vi "Configure.vi"(8 "error in":errorcluster, 10 "ConfigRef In":T1, 11 "HH802U in":refnum<class "HH802U.lvclass">) -> (0 "error out":errorcluster, 3 "HH802U out":refnum<class "HH802U.lvclass">)   [LabVIEW 2015, in "HH802U.lvclass"]
uses:
  HH802U.lvclass
  <vilib>/Utility/config.llb/Config Data RefNum.ctl
  HH802U.lvclass/HH802U.ctl
  <vilib>/Utility/config.llb/Read Key (String).vi
  <vilib>/Utility/config.llb/Read Key (U32).vi
  <vilib>/Instr/_visa.llb/VISA Configure Serial Port (Instr).vi
  <vilib>/Utility/config.llb/NI_LVConfig.lvlib
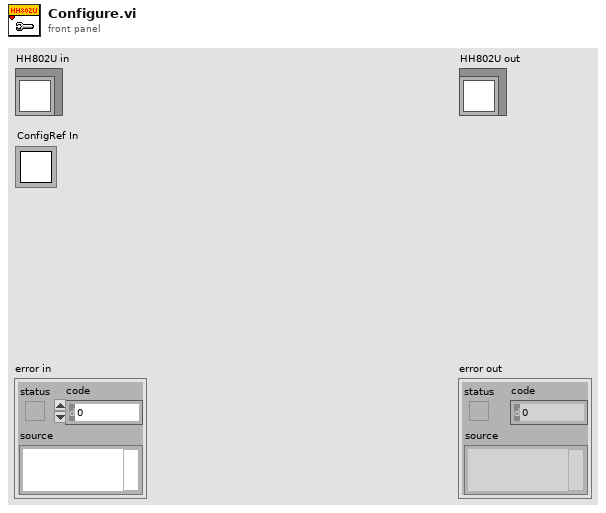
[diagram p1: front panel]
types:
  T1 = typedef "NI_LVConfig.lvlib/Config Data RefNum.ctl" = refnum<k1>
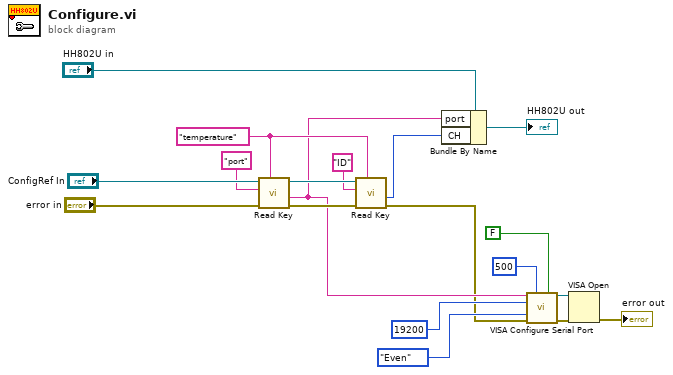
[diagram p0: block diagram]
diagram:
  w8 = "temperature" ("section")
  n1 = call-poly <vilib>:"Read Key.vi"("section"=w8, "error in (no error)"="error in", "key"="port", "refnum"="ConfigRef In") -> ("error out"=w9:errorcluster, "value"=w4:string, "refnum out"=w10:T1)  [unwired: 4 in, 1 out]
  n2 = call-poly <vilib>:"Read Key.vi"("section"=w8, "error in (no error)"=w9, "key"="ID", "refnum"=w10) -> ("error out"=w2:errorcluster, "value"=w3:u32)  [unwired: 4 in, 2 out]
  n3 = Bundle By Name(cluster="HH802U in", "port"=w4, "CH"=w3) -> (→"HH802U out":refnum<class "HH802U.lvclass">)
  n4 = call-poly "VISA Configure Serial Port"("VISA resource name"=w4, "timeout (10sec)"=u32 500, "Enable Termination\nChar (T)"=FALSE ("Enable Termination\nChar (T)"), "baud rate (9600)"=u32 19200, "parity (0:none)"=enum16{"None", "Odd", "Even", "Mark", "Space"}."Even", "error in (no error)"=w2) -> ("VISA resource name out"=w14:refnum<visa-resource-name>, "error out"=w13:errorcluster)  [unwired: 8 in]
  n5 = VISA Open(error in (no error)=w13, VISA resource name=w14) -> (error out=→"error out":errorcluster)  [unwired: 3 in, 1 out]
